vi "Get Number New Images.vi"(10 "last":i32, 11 "first":i32) -> (1 "function return":u32, 2 "last out":i32, 3 "first out":i32)   [LabVIEW 2018, in "AndorSDK.lvlib"]
doc: "EXPNETTYPE unsigned int WINAPI GetNumberNewImages(long * first, long * last);"
uses:
  AndorSDK.lvlib
  ATMCD32D.dll
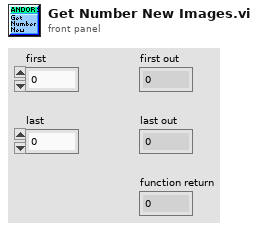
[diagram p1: front panel]
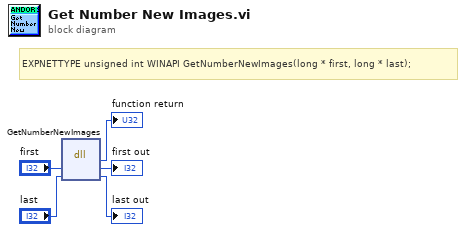
[diagram p0: block diagram]
diagram:
  # "EXPNETTYPE unsigned int WINAPI GetNumberNewImages(long * first, long * last);"
  n1 = dll-call lib="PTH2babs E\nPersönliches02 - Arbeit03-HiwijobsLabviewCodelibANDOR\tAndor SDK\nATMCD32D.*" fn="GetNumberNewImages"("first"="first", "last"="last") -> (→"function return":u32, "first"=→"first out":i32, "last"=→"last out":i32)  [unwired: 3 in, 2 out]
